vi "Initialize Modules.vi"(8 "error in (no error)":errorcluster, 10 "Modules":refnum<class "Module.lvclass">[](array[class]), 11 "Block Diagram in":refnum<class "VI.lvclass">) -> (0 "error out":errorcluster, 3 "Block Diagram out":refnum<class "VI.lvclass">)   [LabVIEW 2015, in "VI.lvclass"]
uses:
  VI.lvclass
  Module/Module/Module.lvclass
  VI.lvclass/VI.ctl
  Main Sequence/Main Sequence.lvclass
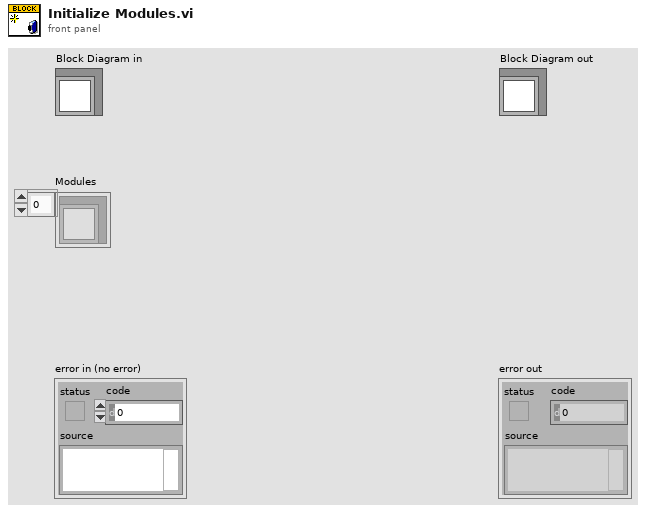
[diagram p1: front panel]
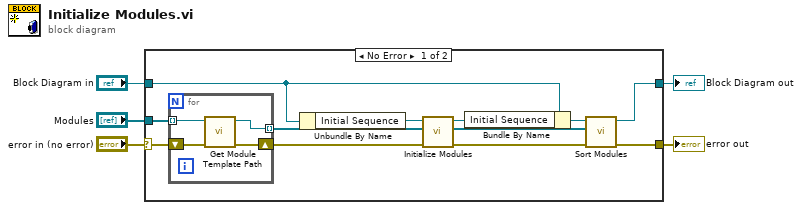
[diagram p0: block diagram]
diagram:
  n1 = case shown="No Error" "error in (no error)" {
    selector: "error in (no error)" -> [w15 w23]
    tunnel: [w12 w23] -> w4
    tunnel: [w10 w22] -> w2
    tunnel: "Block Diagram in" -> [w7 w22]
    tunnel: "Modules" -> [w16 _]
    frame No Error {
      n2 = for {
        tunnel: w16 -> [w18] mode=indexing
        tunnel: [w21] -> w11 mode=indexing
        shift-right: [w20] -> w14
        shift-left: w15 -> [w19]
        n3 = call-dynamic "Get Module Template Path.vi"("error in (no error)"=w19, "Module in"=w18) -> ("error out"=w20:errorcluster, "Module out"=w21:refnum<class "Module.lvclass">)  [unwired: 8 in]
      }
      n4 = Unbundle By Name(w7) -> ("Initial Sequence"=w17:refnum<class "Main Sequence.lvclass">)
      n5 = call "Initialize Modules.vi"("error in (no error)"=w14, "Modules"=w11, "Initial Sequence in"=w17) -> ("error out"=w13:errorcluster, "Modules"=w9:refnum<class "Module.lvclass">[], "Initial Sequence out"=w8:refnum<class "Main Sequence.lvclass">)  [unwired: 6 in]
      n6 = Bundle By Name(cluster=w7, "Initial Sequence"=w8) -> (w6:refnum<class "VI.lvclass">)
      n7 = call "Sort Modules.vi"("error in (no error)"=w13, "Modules"=w9, "Block Diagram in"=w6) -> ("error out"=w12:errorcluster, "Block Diagram out"=w10:refnum<class "VI.lvclass">)  [unwired: 7 in]
    }
    frame Error {
    }
  }
  "error out" <- w4
  "Block Diagram out" <- w2
